vi "FGV사용예.vi"() -> ()   [LabVIEW 2020]
panel:
  out "수신":dbl
  out "송신":dbl
  in  "정지 2":bool
  in  "정지":bool
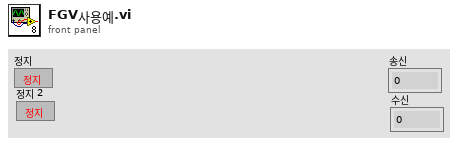
[diagram p1: front panel]
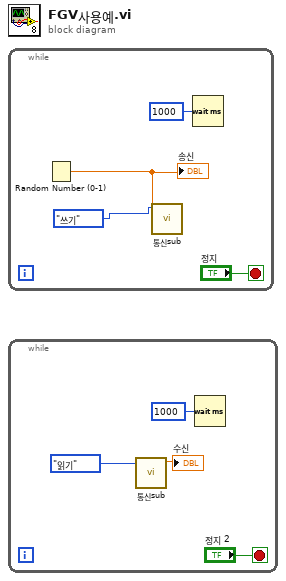
[diagram p0: block diagram]
diagram:
  n1 = while {
    stop <- "정지" stop-if-true
    n2 = Random Number (0-1)() -> (number: 0 to 1=w1:dbl)
    "송신" <- w1
    n3 = call "통신sub.vi"("FGV 상태"=enum16{"쓰기", "읽기", ""}."쓰기", "입력"=w1) -> ()  [unwired: 8 in, 1 out]
    n4 = Wait (ms)(milliseconds to wait=u32 1000 ("대기 시간 (ms)")) -> ()  [unwired: 1 out]
  }
  n5 = while {
    stop <- "정지 2" stop-if-true
    n6 = call "통신sub.vi"("FGV 상태"=enum16{"쓰기", "읽기", ""}."읽기") -> ("출력"=→"수신":dbl)  [unwired: 9 in]
    n7 = Wait (ms)(milliseconds to wait=u32 1000 ("대기 시간 (ms)")) -> ()  [unwired: 1 out]
  }
